vi "1s pulse creator.vi"(10 "input":bool) -> (2 "output":bool)   [LabVIEW 2019]
uses:
  <vilib>/measure/mamon.llb/Trigger Detection for 1 Channel.vi
  <vilib>/measure/NI_MAPro.lvlib
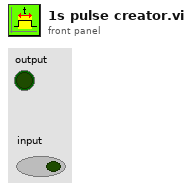
[diagram p1: front panel]
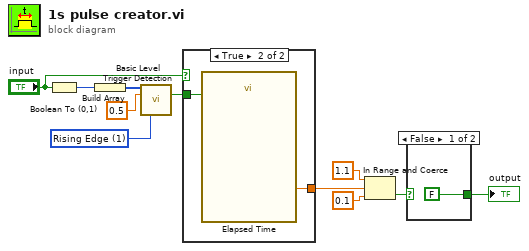
[diagram p0: block diagram]
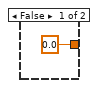
[diagram p2: hidden frame]
diagram:
  w3 = u16 1 items=["Falling Edge", "Rising Edge"] ("trigger slope")
  n1 = Boolean To (0,1)(Boolean="input") -> (0, 1=w6:i16)
  n2 = Build Array(w6) -> (w5:i16[])
  n3 = call-poly <vilib>:"Basic Level Trigger Detection.vi"("signal in"=w5, "level"=0.5, "trigger slope"=w3) -> ("trigger detected?"=w2:bool)  [unwired: 10 in, 2 out]
  n4 = case shown="True" "input" {
    tunnel: [0.0 ("Elapsed Time (s)") w13] -> w11
    tunnel: w2 -> [_ w14]
    frame False {
    }
    frame True {
      n5 = call "Elapsed Time"("Reset"=w14) -> ("Elapsed Time (s)"=w13:dbl)  [unwired: 11 in, 7 out]
    }
  }
  n6 = In Range and Coerce(upper limit=1.1, x=w11, lower limit=0.1) -> (In Range?=w8:bool)  [unwired: 1 out]
  n7 = case shown="False" w8 {
    selector: w8 -> [_ w16]
    tunnel: [FALSE w16] -> w7
    frame False {
    }
    frame True {
    }
  }
  "output" <- w7
